vi "read_counter.vi"() -> ()   [LabVIEW 2009]
uses:
  <vilib>/DAQmx/create/channels.llb/DAQmx Create Channel (CI-Count Edges).vi
  <vilib>/DAQmx/read.llb/DAQmx Read (Counter DBL 1Chan 1Samp).vi
  Program Files/National Instruments/LabVIEW 2009/resource/objmgr/daqmx.rc
panel:
  out "Waveform Chart":i32(graph)
  out "x-y":i32
  in  "Terminal":tag="/Dev1/PFI0"
  in  "counter":tag="Dev1/ctr0"
  out "Meter":dbl(knob) scale=0.0..10000.0
  out "Counts/sec":dbl
  in  "milliseconds to count for":i32=100
  in  "stop":bool
  out "Counts total":i32
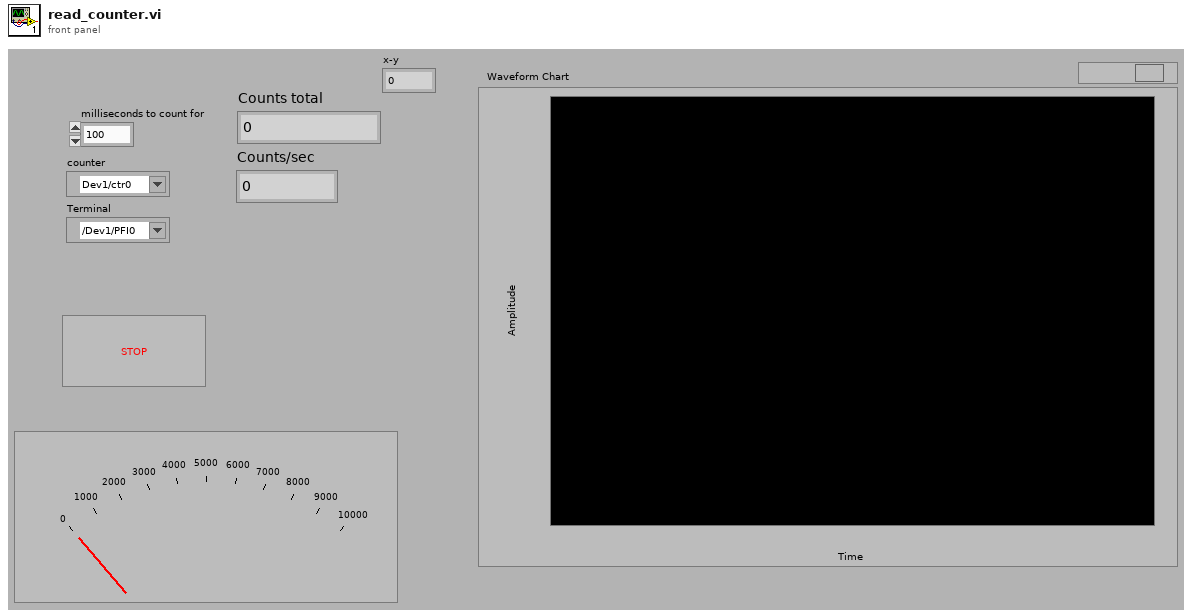
[diagram p1: front panel]
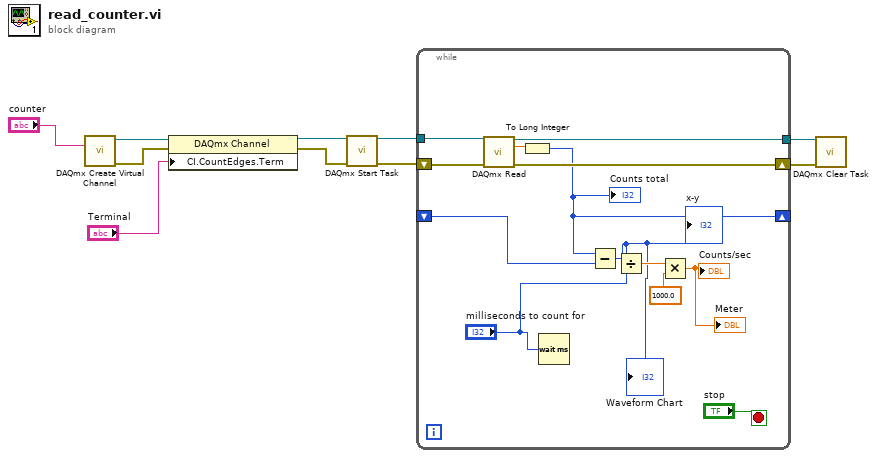
[diagram p0: block diagram]
diagram:
  n1 = call-poly <vilib>:"DAQmx Create Virtual Channel.vi"("counter"="counter") -> ("task out"=w10:refnum<k21>, "error out"=w8:errorcluster)  [unwired: 13 in]
  n2 = property class="DAQmx Channel"(reference=w10, error in=w8, "CI.CountEdges.Term"="Terminal") -> (reference out=w5:refnum<k21>, error out=w4:errorcluster)
  n3 = call <vilib>:"DAQmx Start Task.vi"("task/channels in"=w5, "error in"=w4) -> ("task out"=w3:refnum<k21>, "error out"=w2:errorcluster)  [unwired: 12 in]
  n4 = while {
    shift-right: [w23] -> w6
    shift-left: w2 -> [w22]
    tunnel: [w21] -> w7
    tunnel: w3 -> [w19]
    shift-right: [w13] -> _
    shift-left: _ -> [w18]
    stop <- "stop" stop-if-true
    n5 = call-poly <vilib>:"DAQmx Read.vi"("task/channels in"=w19, "error in"=w22) -> ("task out"=w21:refnum<k21>, "data"=w14:dbl, "error out"=w23:errorcluster)  [unwired: 11 in]
    n6 = To Long Integer(number=w14) -> (32bit integer=w13:i32)
    "Counts total" <- w13
    n7 = Wait (ms)(milliseconds to wait="milliseconds to count for") -> ()  [unwired: 1 out]
    n8 = Subtract(x=w13, y=w18) -> (x-y=w11:i32)
    "x-y" <- w11
    "Waveform Chart" <- w11
    n9 = Divide(x=w11, y="milliseconds to count for") -> (x/y=w16:dbl)
    n10 = Multiply(x=w16, y=1000.0) -> (x*y=→"Counts/sec" →"Meter":dbl)
  }
  n11 = call <vilib>:"DAQmx Clear Task.vi"("task in"=w7, "error in"=w6) -> ()  [unwired: 13 in, 1 out]
